vi "Close Device.vi"(0 "Register Bus":T1, 11 "error in":errorcluster) -> (4 "fpga ref":refnum<k20>, 15 "error out":errorcluster)   [LabVIEW 2017]
doc: "Close the register bus to the device.\n\n<B>Input Parameters</B>\n\n<B>Register Bus</B> The Register Bus object created by the ni579x Open VI and used as the session handle for the NI-579x Configuration Design Library.\n\n<B>error in</B> describes error conditions that occur before this node runs. This input provides standard 'error in' functionality.\n\n<B>Output Parameters</B>\n\n<B>fpga ref</B> is the (open) FPGA reference to the device.\n\n<B>error out</B> contains error information. This output provides standard 'error out' functionality."
uses:
  <instrlib>/_niInstr/Register Bus/v0/Host/Public/Register Bus Session.ctl
  <instrlib>/_niInstr/Register Bus/v0/Host/Private/Session Data.ctl
  <instrlib>/ni579x/Config/v2/Host/ni579x Config v2 Host.lvlib
  <instrlib>/_niInstr/Register Bus/v0/Host/niInstr Register Bus v0 Host.lvlib
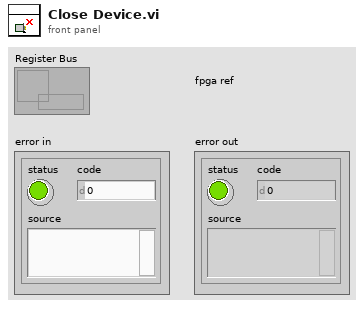
[diagram p1: front panel]
types:
  T1 = typedef "niInstr Register Bus v0 Host.lvlib/Register Bus Session.ctl" = refnum<queue>
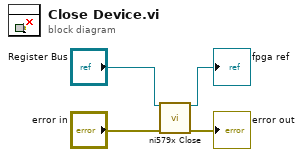
[diagram p0: block diagram]
diagram:
  n1 = call <instrlib>:"ni579x Close.vi"("Register Bus"="Register Bus", "error in"="error in") -> ("fpga ref"=→"fpga ref":refnum<k20>, "error out"=→"error out":errorcluster)  [unwired: 12 in]
